vi "Get pos axis.vi"(8 "error in (no error)":errorcluster, 10 "Axis":i32=1 min=1 max=4, 11 "OWIS_TANGO in":refnum<class "OWIS_TANGO.lvclass">) -> (0 "error out":errorcluster, 2 "Pos":dbl, 3 "OWIS_TANGO out":refnum<class "OWIS_TANGO.lvclass">)   [LabVIEW 2020, in "OWIS_TANGO.lvclass"]
uses:
  OWIS_TANGO.lvclass
  OWIS_TANGO.lvclass/OWIS_TANGO.ctl
  tango-binding-3.0.0-for-labview-2014-windows-x64/vis/tango_vi.llb/_TangoReadDoubleScalarAttribute.vi
  tango-binding-3.0.0-for-labview-2014-windows-x64/vis/tango_vi.llb/tango.lvlib
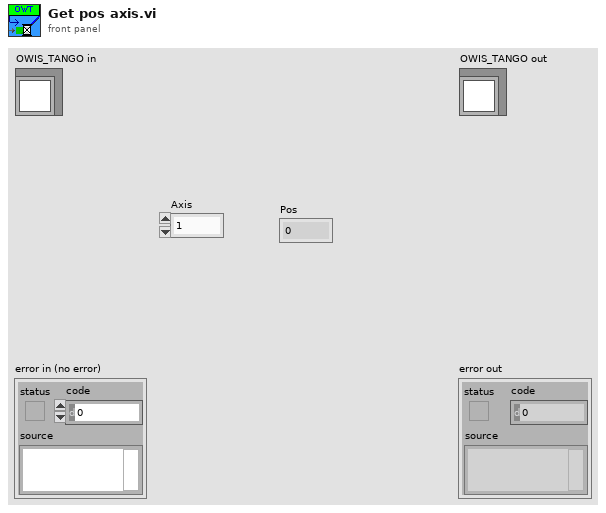
[diagram p1: front panel]
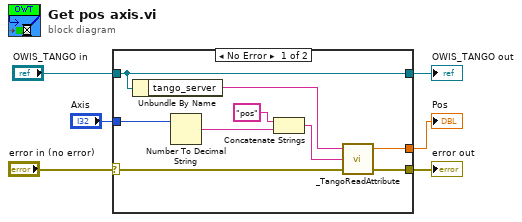
[diagram p0: block diagram]
diagram:
  n1 = case shown="No Error" "error in (no error)" {
    selector: "error in (no error)" -> [w14 w17]
    tunnel: [w15 w17] -> w5
    tunnel: "OWIS_TANGO in" -> [w8 w16]
    tunnel: "Axis" -> [w12 _]
    tunnel: [w8 w16] -> w2
    tunnel: [w9 _] -> w1
    frame No Error {
      n2 = Unbundle By Name(w8) -> ("tango_server"=w7:string)
      n3 = Number To Decimal String(number=w12) -> (decimal integer string=w11:string)  [unwired: 1 in]
      n4 = Concatenate Strings("pos" ("attribute name"), w11) -> (w10:string)
      n5 = call-poly "_TangoReadAttribute.vi"("error in"=w14, "attribute name"=w10, "device name"=w7) -> ("error out"=w15:errorcluster, "value"=w9:dbl)  [unwired: 1 out]
    }
    frame Error {
    }
  }
  "error out" <- w5
  "OWIS_TANGO out" <- w2
  "Pos" <- w1
